vi "PressurizedTube.vi"(7 "Pipe Network Parameters":T2, 8 "Unused Output (mB/t)":i64, 9 "Push Input (mB/t)":i64) -> (0 "Rejected Input (mB/t)":i64, 1 "Output (mB/t)":i64, 3 "Buffered (mB)":i64, 4 "Buffer Size (mB)":i64)   [LabVIEW 2023]
uses:
  Tier.ctl
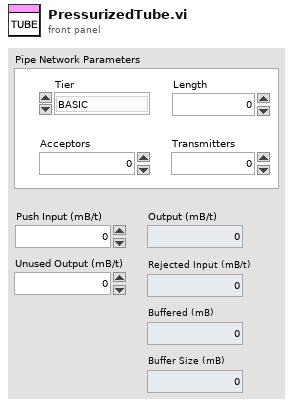
[diagram p1: front panel]
types:
  T1 = typedef "Tier.ctl" = enum16{"BASIC", "ADVANCED", "ELITE", "ULTIMATE"}
  T2 = cluster{"Tier":T1, "Acceptors":i64, "Length":i64, "Transmitters":i64}
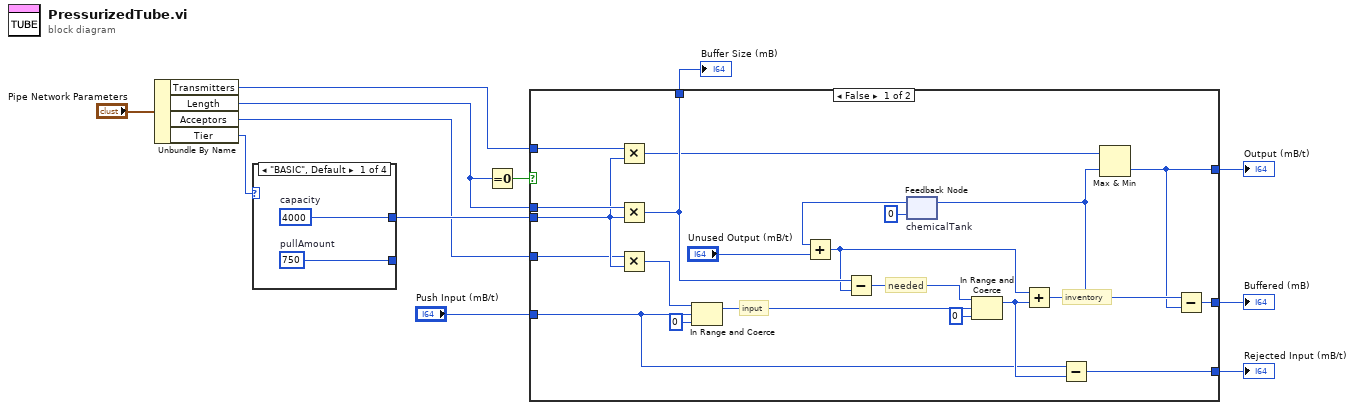
[diagram p0: block diagram]
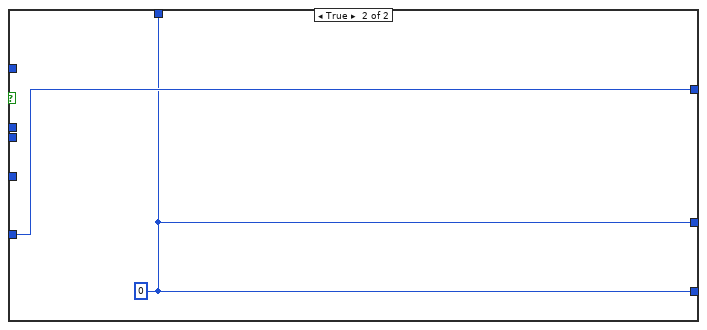
[diagram p2: hidden frame]
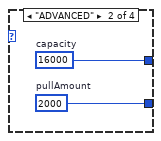
[diagram p3: hidden frame]
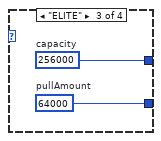
[diagram p4: hidden frame]
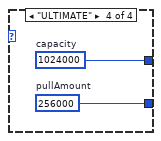
[diagram p5: hidden frame]
diagram:
  n1 = Unbundle By Name("Pipe Network Parameters") -> ("Transmitters"=w1:i64, "Length"=w3:i64, "Acceptors"=w2:i64, "Tier"=w4:T1)
  n2 = case shown="\"BASIC\", Default" w4 {
    tunnel: [w14 w16 w18 w20] -> w11
    tunnel: [w13 w15 w17 w19] -> _
    frame "BASIC", Default {
      w13 = i64 750  # pullAmount
      w14 = i64 4000  # capacity
    }
    frame "ADVANCED" {
      w15 = i64 2000  # pullAmount
      w16 = i64 16000  # capacity
    }
    frame "ELITE" {
      w17 = i64 64000  # pullAmount
      w18 = i64 256000  # capacity
    }
    frame "ULTIMATE" {
      w19 = i64 256000  # pullAmount
      w20 = i64 1024000  # capacity
    }
  }
  n3 = Equal To 0?(x=w3) -> (x = 0?=w7:bool)
  n4 = case shown="False" w7 {
    tunnel: w3 -> [w41 _]
    tunnel: [w38 w42] -> w12
    tunnel: w11 -> [w37 _]
    tunnel: [w33 w42] -> w10
    tunnel: [w26 w42] -> w9
    tunnel: [w25 w43] -> w8
    tunnel: "Push Input (mB/t)" -> [w23 w43]
    tunnel: w2 -> [w22 _]
    tunnel: w1 -> [w21 _]
    frame False {
      # "inventory"
      # "needed"
      # "input"
      n5 = Multiply(x=w21, y=w37) -> (x*y=w28:i64)
      n6 = Multiply(x=w41, y=w37) -> (x*y=w33:i64)
      n7 = Multiply(x=w22, y=w37) -> (x*y=w40:i64)
      n8 = In Range and Coerce(upper limit=w40, x=w23, lower limit=i64 0) -> (coerced(x)=w39:i64)  [unwired: 1 out]
      n9 = feedback #1 "chemicalTank"(i64 0) -> (w36:i64)
      n10 = Add(x=w36, y="Unused Output (mB/t)") -> (x+y=w30:i64)
      n11 = Subtract(x=w33, y=w30) -> (x-y=w32:i64)
      n12 = In Range and Coerce(upper limit=w32, x=w39, lower limit=i64 0) -> (coerced(x)=w29:i64)  [unwired: 1 out]
      n13 = Add(x=w30, y=w29) -> (x+y=w27:i64)
      n14 = feedback-in #1(w27) -> ()
      n15 = Subtract(x=w23, y=w29) -> (x-y=w38:i64)
      n16 = Max & Min(x=w28, y=w27) -> (min(x,y)=w25:i64)  [unwired: 1 out]
      n17 = Subtract(x=w27, y=w25) -> (x-y=w26:i64)
    }
    frame True {
      w42 = i64 0
    }
  }
  "Rejected Input (mB/t)" <- w12
  "Buffer Size (mB)" <- w10
  "Output (mB/t)" <- w8
  "Buffered (mB)" <- w9
